vi "Run Step.vi"(8 "error in (no error)":errorcluster, 9 "result allocation":T1, 10 "parameters":T1, 11 "Wait On Boolean Step in":refnum<class "Wait On Boolean Step.lvclass">) -> (0 "error out":errorcluster, 1 "results":T1, 2 "parameter allocation":T1, 3 "Wait On Boolean Step out":refnum<class "Wait On Boolean Step.lvclass">)   [LabVIEW 2015, in "Wait On Boolean Step.lvclass"]
uses:
  Wait On Boolean Step.lvclass
  <vilib>/NI/Tag Bus/table/data table.ctl
  Wait On Boolean Step.lvclass/Wait On Boolean Step.ctl
  classes/Step/Execution/StepState.ctl
  classes/Step/Execution/Step Status.ctl
  classes/Step/Execution/Step Flow Control.ctl
  <vilib>/NI/Tag Bus/table/data polymorphs/read one/read Boolean.vi
  Write Timer Value (ms).vi
  <vilib>/NI/Tag Bus/table/data table.lvlib
  classes/Step/Execution/Step.lvclass
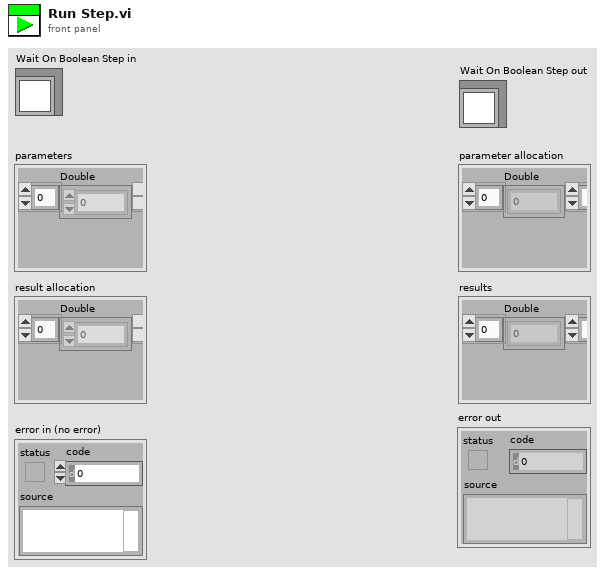
[diagram p1: front panel]
types:
  T1 = typedef "tag bus.lvlib/data table.lvlib/data table.ctl" = cluster{"Double":dbl[], "Single":sgl[], "I64":i64[], "I32":i32[], "I16":i16[], "I8":i8[], "U64":u64[], "U32":u32[], "U16":u16[], "U8":u8[], "Boolean":bool[], "String":string[], "Array of Double":cluster{"DBL Array":dbl[]}[], "Array of Single":cluster{"SGL Array":sgl[]}[], "Array of I64":cluster{"I64 Array":i64[]}[], "Array of I32":cluster{"I32 Array":i32[]}[], "Array of I16":cluster{"I16 Array":i16[]}[], "Array of I8":cluster{"I8 Array":i8[]}[], "Array of U64":cluster{"U64 Array":u64[]}[], "Array of U32":cluster{"U32 Array":u32[]}[], "Array of U16":cluster{"U16 Array":u16[]}[], "Array of U8":cluster{"U8 Array":u8[]}[], "Array of Boolean":cluster{"Boolean Array":bool[]}[], "Array of String":cluster{"String Array":string[]}[]}
  T2 = typedef "Step.lvclass/StepState.ctl" = cluster{"Step State":T3, "Flow Control":T4, "Jump Index":i32, "Done":bool}
  T3 = typedef "Step.lvclass/Step Status.ctl" = enum16{"Start", "Passed", "Failed", "Error", "Done", "Terminated", "Skipped", "Running"}
  T4 = typedef "Step.lvclass/Step Flow Control.ctl" = enum16{"Next Step", "Jump"}
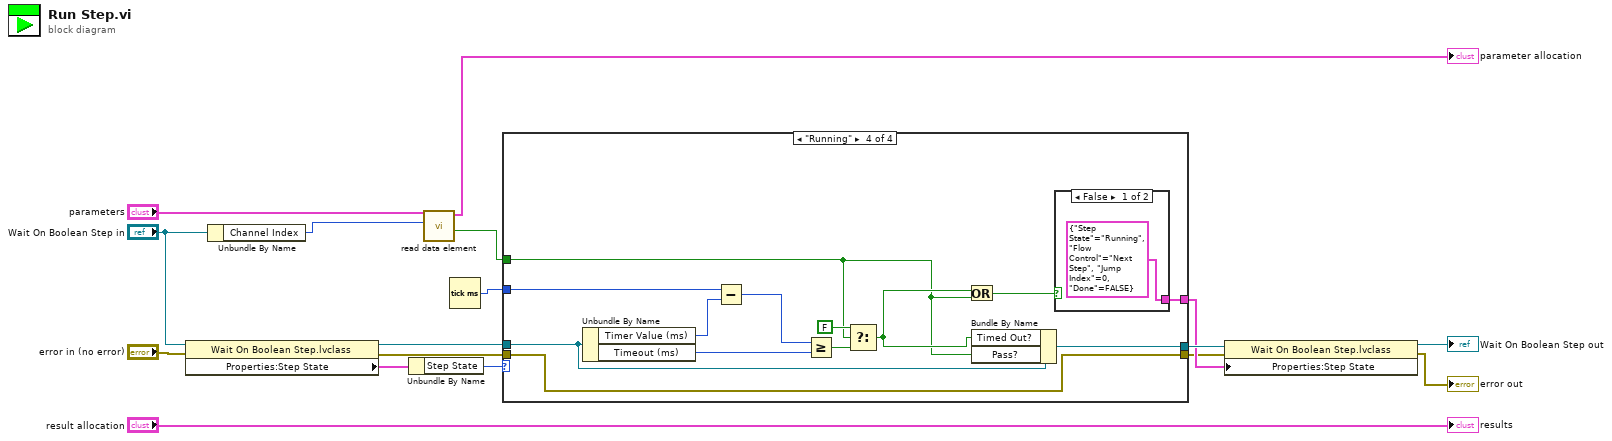
[diagram p0: block diagram]
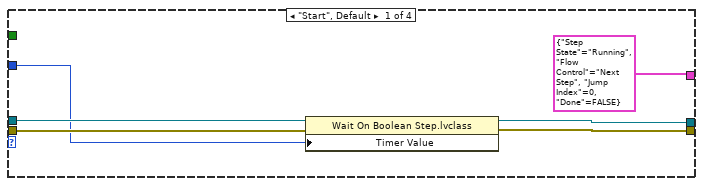
[diagram p2: hidden frame]
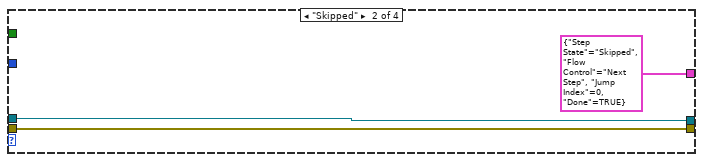
[diagram p3: hidden frame]
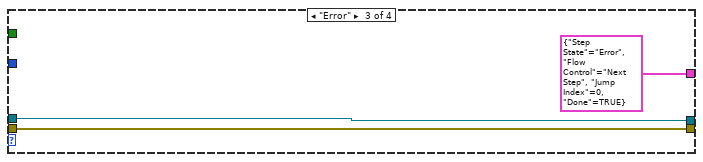
[diagram p4: hidden frame]
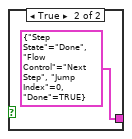
[diagram p5: hidden frame]
diagram:
  n1 = property class="Wait On Boolean Step.lvclass"(reference="Wait On Boolean Step in", error in="error in (no error)") -> (reference out=w15:refnum<class "Wait On Boolean Step.lvclass">, error out=w14:errorcluster, "Properties:Step State"=w17:T2)
  n2 = Unbundle By Name("Wait On Boolean Step in") -> ("Channel Index"=w8:i32)
  n3 = Unbundle By Name(w17) -> ("Step State"=w16:T3)
  n4 = call-poly <vilib>:"read data element.vi"("index"=w8, "data table in"="parameters") -> ("value"=w9:bool, "data table out"=→"parameter allocation":T1)  [unwired: 8 in]
  n5 = Tick Count (ms)() -> (millisecond timer value=w11:u32)
  n6 = case shown="\"Running\"" w16 {
    tunnel: w15 -> [w22 w25 w28 w38]
    tunnel: w14 -> [w23 w26 w29 w36]
    tunnel: [w21 w25 w28 w37] -> w5
    tunnel: w11 -> [w20 _ _ w41]
    tunnel: w9 -> [_ _ _ w32]
    tunnel: [w19 w26 w29 w36] -> w3
    tunnel: [T2 {"Step State"=enum."Running", "Flow Control"=enum."Next Step", "Jump Index"=0, "Done"=FALSE} ("Step State") T2 {"Step State"=enum."Skipped", "Flow Control"=enum."Next Step", "Jump Index"=0, "Done"=TRUE} ("Step State") T2 {"Step State"=enum."Error", "Flow Control"=enum."Next Step", "Jump Index"=0, "Done"=TRUE} ("Step State") w30] -> w4
    frame "Start", Default {
      n7 = property class="Wait On Boolean Step.lvclass"(reference=w22, error in=w23, "Timer Value"=w20) -> (reference out=w21:refnum<class "Wait On Boolean Step.lvclass">, error out=w19:errorcluster)
    }
    frame "Skipped" {
    }
    frame "Error" {
    }
    frame "Running" {
      n8 = Unbundle By Name(w38) -> ("Timer Value (ms)"=w42:i32, "Timeout (ms)"=w39:i32)
      n9 = Subtract(x=w41, y=w42) -> (x-y=w40:u32)
      n10 = Greater Or Equal?(x=w40, y=w39) -> (x >= y?=w34:bool)
      n11 = Select(t=FALSE ("value"), s=w32, f=w34) -> (s? t:f=w33:bool)
      n12 = Or(x=w33, y=w32) -> (x .or. y?=w31:bool)
      n13 = Bundle By Name(cluster=w38, "Timed Out?"=w33, "Pass?"=w32) -> (w37:refnum<class "Wait On Boolean Step.lvclass">)
      n14 = case shown="False" w31 {
        tunnel: [T2 {"Step State"=enum."Running", "Flow Control"=enum."Next Step", "Jump Index"=0, "Done"=FALSE} ("Step State") T2 {"Step State"=enum."Done", "Flow Control"=enum."Next Step", "Jump Index"=0, "Done"=TRUE} ("Step State")] -> w30
        frame False {
        }
        frame True {
        }
      }
    }
  }
  n15 = property class="Wait On Boolean Step.lvclass"(reference=w5, error in=w3, "Properties:Step State"=w4) -> (reference out=→"Wait On Boolean Step out":refnum<class "Wait On Boolean Step.lvclass">, error out=→"error out":errorcluster)
  "results" <- "result allocation"
